vi "Init.vi"(8 "error in":errorcluster, 9 "Format Specifier":string="%s - %-7s - %s - %s - %d - %s", 10 "Datetime format":string="%Y-%m-%d %H:%M:%S", 11 "Formatter in":refnum<class "Formatter.lvclass">) -> (0 "error out":errorcluster, 3 "Formatter out":refnum<class "Formatter.lvclass">)   [LabVIEW 2024, in "hse-logger.lvlib" / "Formatter.lvclass"]
doc: "____\nHAMPEL SOFTWARE ENGINEERING v2.2.2 (2025-01-16 15:41)"
uses:
  <vilib>/Hampel Software Engineering/HSE Logger/Formatter/Formatter.lvclass
  <vilib>/Hampel Software Engineering/HSE Logger/Formatter/Formatter.lvclass/Formatter.ctl
panel:
  # "Time - Level - Callchain - Message - Error Code - Error Message"
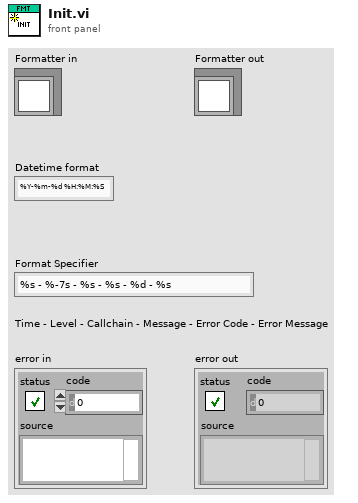
[diagram p1: front panel]
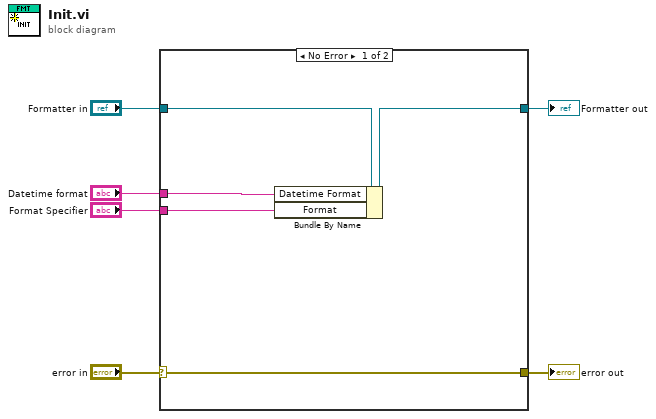
[diagram p0: block diagram]
diagram:
  n1 = case shown="No Error" "error in" {
    selector: "error in" -> [w11 w13]
    tunnel: [w11 w13] -> w5
    tunnel: [w9 w12] -> w3
    tunnel: "Formatter in" -> [w10 w12]
    tunnel: "Datetime format" -> [w8 _]
    tunnel: "Format Specifier" -> [w7 _]
    frame No Error {
      n2 = Bundle By Name(cluster=w10, "Datetime Format"=w8, "Format"=w7) -> (w9:refnum<class "Formatter.lvclass">)
    }
    frame Error {
    }
  }
  "error out" <- w5
  "Formatter out" <- w3
